vi "Check if configuration files exist.vi"(8 "error in (no error)":errorcluster, 11 "TemplateBase in":refnum<class "Cobolt.lvclass">) -> (0 "error out":errorcluster, 2 "configuration file exists?":bool, 3 "TemplateBase out":refnum<class "Cobolt.lvclass">)   [LabVIEW 2012, in "Cobolt.lvclass"]
doc: "Checks whether all required configuration files for the component exist."
uses:
  Cobolt.lvclass
  <vilib>/Distrio/Murmex/Murmex/Murmex.lvclass
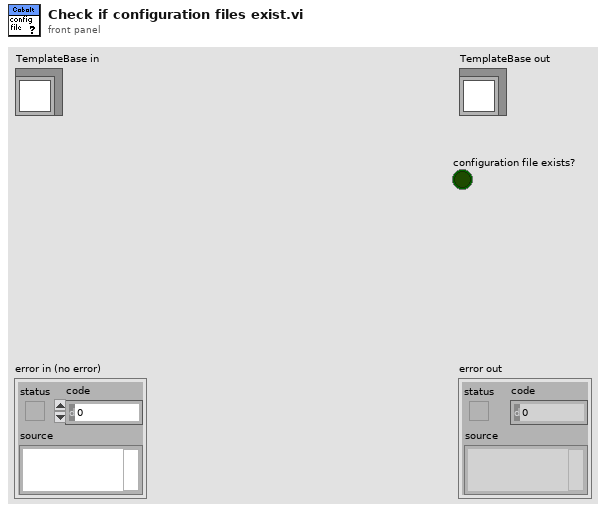
[diagram p1: front panel]
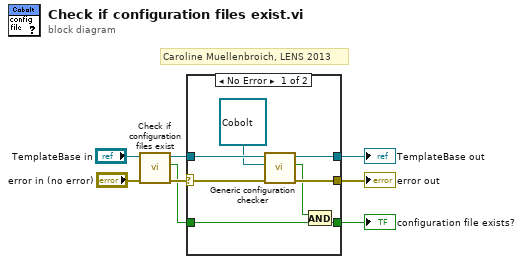
[diagram p0: block diagram]
diagram:
  # "Caroline Muellenbroich, LENS 2013"
  n1 = call-parent "Check if configuration files exist.vi"("error in (no error)"="error in (no error)", "MurmexBase in"="TemplateBase in") -> ("error out"=w6:errorcluster, "configuration file exists?"=w2:bool, "MurmexBase out"=w5:refnum<class "Cobolt.lvclass">)  [unwired: 7 in]
  n2 = case shown="No Error" w6 {
    selector: w6 -> [w16 w19]
    tunnel: [w14 w19] -> w4
    tunnel: [w13 w18] -> w3
    tunnel: w5 -> [w15 w18]
    tunnel: w2 -> [w11 w17]
    tunnel: [w9 w17] -> w1
    frame No Error {
      n3 = call <vilib>:"Generic configuration checker.vi"("error in (no error)"=w16, "inheritance level"=refnum<class "Cobolt.lvclass"> refnum ("Template.lvclass"), "Murmex in"=w15) -> ("error out"=w14:errorcluster, "configuration file exists?"=w10:bool, "Murmex out"=w13:refnum<class "Cobolt.lvclass">)  [unwired: 6 in]
      n4 = And(x=w10, y=w11) -> (x .and. y?=w9:bool)
    }
    frame Error {
    }
  }
  "error out" <- w4
  "TemplateBase out" <- w3
  "configuration file exists?" <- w1
